vi "DealWithScrollbars.vi"(8 "error in (no error)":errorcluster, 11 "Tree":refnum<vi>) -> (0 "error out":errorcluster)   [LabVIEW 2021]
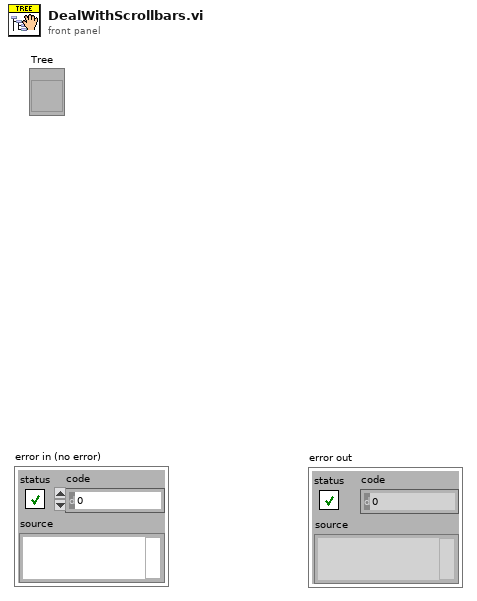
[diagram p1: front panel]
types:
  T1 = enum16{"User-specified Font", "Application Font", "System Font", "Dialog Font"}
  T2 = typedef "LVPositionTypeDef.ctl" = cluster{"Left":i32, "Top":i32}
  T3 = cluster{"left":i16, "top":i16, "right":i16, "bottom":i16}
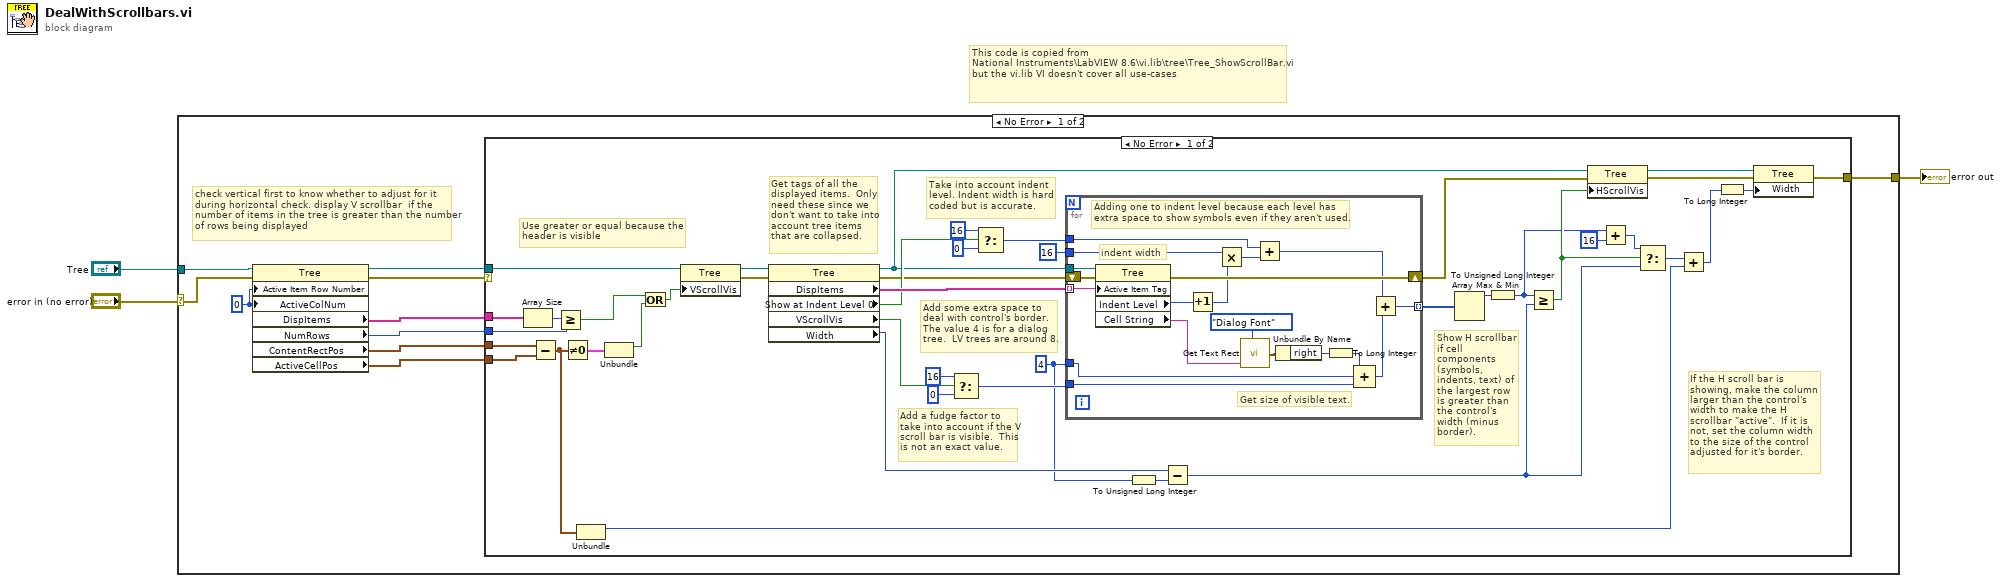
[diagram p0: block diagram]
diagram:
  # "This code is copied from \nNational Instruments\\LabVIEW 8.6\\vi.lib\\tree\\Tree_ShowScrollBar.vi but the vi.lib VI doesn't cover all use-cases"
  n1 = case shown="No Error" "error in (no error)" {
    selector: "error in (no error)" -> [w10 w76]
    tunnel: "Tree" -> [w11 _]
    tunnel: [w9 w76] -> w1
    frame No Error {
      w5 = 0 ("Active Cell:Active Column Number")
      # "check vertical first to know whether to adjust for it during horizontal check. display V scrollbar  if the number of items in the tree is greater than the number of rows being displayed"
      n2 = property class="Tree"(reference=w11, error in=w10, "Active Item Row Number"=w5, "ActiveColNum"=w5) -> (reference out=w13:refnum<vi>, error out=w4:errorcluster, "DispItems"=w8:string[], "NumRows"=w12:u32, "ContentRectPos"=w7:T2, "ActiveCellPos"=w6:T2)
      n3 = case shown="No Error" w4 {
        tunnel: w13 -> [w32 _]
        tunnel: w12 -> [w31 _]
        tunnel: [w26 _] -> w9
        tunnel: w8 -> [w22 _]
        tunnel: w7 -> [w21 _]
        tunnel: w6 -> [w20 _]
        frame No Error {
          w38 = 4 ("contorl border width")
          # "Use greater or equal because the\nheader is visible"
          # "If the H scroll bar is showing, make the column larger than the control's width to make the H scrollbar \"active\".  If it is not, set the column width to the size of the control adjusted for it's border."
          # "Show H scrollbar if cell components (symbols, indents, text) of the largest row is greater than  the control's width (minus border)."
          # "Add some extra space to deal with control's border.  The value 4 is for a dialog tree.  LV trees are around 8."
          # "Take into account indent level. Indent width is hard coded but is accurate."
          # "Add a fudge factor to take into account if the V scroll bar is visible.  This is not an exact value."
          # "Get tags of all the displayed items.  Only need these since we don't want to take into account tree items that are collapsed."
          n4 = Array Size(array=w22) -> (size(s)=w34:i32)
          n5 = Subtract(x=w21, y=w20) -> (x-y=w16:T2)
          n6 = Greater Or Equal?(x=w34, y=w31) -> (x >= y?=w33:bool)
          n7 = Not Equal To 0?(x=w16) -> (x != 0?=w19:cluster{"Left":bool, "Top":bool})
          n8 = Unbundle(w16) -> ("Left"=w14:i32)  [unwired: 1 out]
          n9 = Unbundle(w19) -> ("Left"=w17:bool)  [unwired: 1 out]
          n10 = Or(x=w33, y=w17) -> (x .or. y?=w18:bool)
          n11 = property class="Tree"(reference=w32, "VScrollVis"=w18) -> (reference out=w28:refnum<vi>, error out=w27:errorcluster)  [unwired: 1 in]
          n12 = property class="Tree"(reference=w28, error in=w27) -> (reference out=w29:refnum<vi>, error out=w30:errorcluster, "DispItems"=w50:string[], "Show at Indent Level 0"=w44:bool, "VScrollVis"=w43:bool, "Width"=w39:u32)
          n13 = Select(t=16 ("y"), s=w43, f=0) -> (s? t:f=w54:i32)
          n14 = Select(t=16 ("y"), s=w44, f=0) -> (s? t:f=w45:i32)
          n15 = for {
            tunnel: w50 -> [w73] mode=indexing
            tunnel: w29 -> [w75]
            tunnel: [w65] -> w51 mode=indexing
            tunnel: w54 -> [w64]
            tunnel: w45 -> [w63]
            tunnel: 16 ("indent width") -> [w62]
            tunnel: w38 -> [w61]
            shift-right: [w60] -> w48
            shift-left: w30 -> [w74]
            # "Adding one to indent level because each level has extra space to show symbols even if they aren't used."
            # "Get size of visible text."
            # "indent width"
            n16 = property class="Tree"(reference=w75, error in=w74, "Active Item Tag"=w73) -> (error out=w60:errorcluster, "Indent Level"=w68:i32, "Cell String"=w69:string)  [unwired: 1 out]
            n17 = Increment(x=w68) -> (x+1=w59:i32)
            n18 = Multiply(x=w62, y=w59) -> (x*y=w67:i32)
            n19 = call <vilib>:"Get Text Rect.vi"("desired font(Application)"=T1."Dialog Font", "text"=w69) -> ("rect"=w71:T3)  [unwired: 4 in, 3 out]
            n20 = Add(x=w63, y=w67) -> (x+y=w57:i32)
            n21 = Unbundle By Name(w71) -> ("right"=w72:i16)
            n22 = To Long Integer(number=w72) -> (32bit integer=w58:i32)
            n23 = Compound Arithmetic op=ADD(w58, w61, w64) -> (w66:i32)
            n24 = Add(x=w57, y=w66) -> (x+y=w65:i32)
          }
          n25 = To Unsigned Long Integer(number=w38) -> (unsigned 32bit integer=w36:u32)
          n26 = Subtract(x=w39, y=w36) -> (x-y=w37:u32)
          n27 = Array Max & Min(array=w51) -> (max value=w55:i32)  [unwired: 3 out]
          n28 = To Unsigned Long Integer(number=w55) -> (unsigned 32bit integer=w35:u32)
          n29 = Greater Or Equal?(x=w35, y=w37) -> (x >= y?=w42:bool)
          n30 = property class="Tree"(reference=w29, error in=w48, "HScrollVis"=w42) -> (reference out=w25:refnum<vi>, error out=w24:errorcluster)
          n31 = Add(x=w35, y=u32 16) -> (x+y=w41:u32)
          n32 = Select(t=w41, s=w42, f=w37) -> (s? t:f=w40:u32)
          n33 = Add(x=w40, y=w14) -> (x+y=w15:u32)
          n34 = To Long Integer(number=w15) -> (32bit integer=w23:i32)
          n35 = property class="Tree"(reference=w25, error in=w24, "Width"=w23) -> (error out=w26:errorcluster)  [unwired: 1 out]
        }
        frame Error {
        }
      }
    }
    frame Error {
    }
  }
  "error out" <- w1
